vi "GetProjInMem.vi"(8 "error in (no error)":errorcluster, 11 "Ring refnum":refnum<vi>) -> (0 "error out":errorcluster, 3 "Project:Projects[]":refnum<vi>[](array[refnum]))   [LabVIEW 2014, in "CS++MessageMakerMain.lvlib" / "CS++MessageMakerMain.lvclass"]
doc: "Searches for all Projects in memory."
uses:
  CS++MessageMakerMain.lvclass
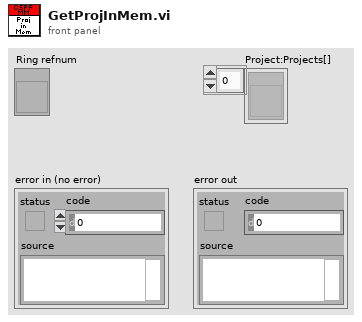
[diagram p1: front panel]
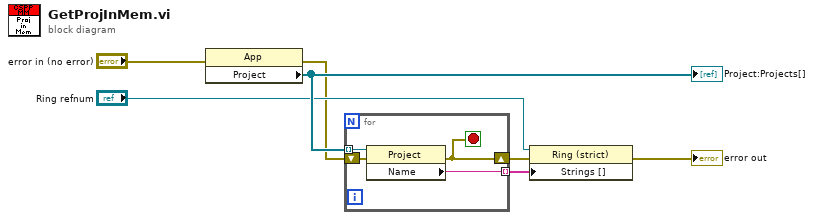
[diagram p0: block diagram]
diagram:
  n1 = property class="App"(error in="error in (no error)") -> (error out=w2:errorcluster, "Project"=w7:refnum<vi>[])  [unwired: 1 in, 1 out]
  "Project:Projects[]" <- w7
  n2 = for {
    tunnel: w7 -> [w11] mode=indexing
    shift-right: [w8] -> w5
    shift-left: w2 -> [w10]
    tunnel: [w9] -> w3 mode=indexing
    stop <- w8 stop-if-true
    n3 = property class="Project"(reference=w11, error in=w10) -> (error out=w8:errorcluster, "Name"=w9:string)  [unwired: 1 out]
  }
  n4 = property class="Ring (strict)"(reference="Ring refnum", error in=w5, "Strings []"=w3) -> (error out=→"error out":errorcluster)  [unwired: 1 out]
